vi "Main.vi"() -> ()   [LabVIEW 2017]
uses:
  <vilib>/Utility/miscctls.llb/LVRowAndColumnTypeDef.ctl
  flow_control/flow_queue_datatype.ctl
  <vilib>/Utility/miscctls.llb/LVPointTypeDef.ctl
  <vilib>/Utility/file.llb/Read Delimited Spreadsheet (string).vi
  <vilib>/Utility/file.llb/Write Delimited Spreadsheet (string).vi
panel:
  out "NG":string
  out "OK":string
  out "STATUS":string
  out "Edit Position":T1
  in  "Save Button":bool
  out "FILE":string[][](array[string])
  out "VISA resource name out":refnum<visa-resource-name>
  out "TESTING":bool
  in  "TEST Button":bool
  in  "Path":path
  out "DEFINE HEADER":string[][](array[string])
  out "Table":string[][](table)
  out "DEFINE IO":string[][](array[string])
  # "FT 4"
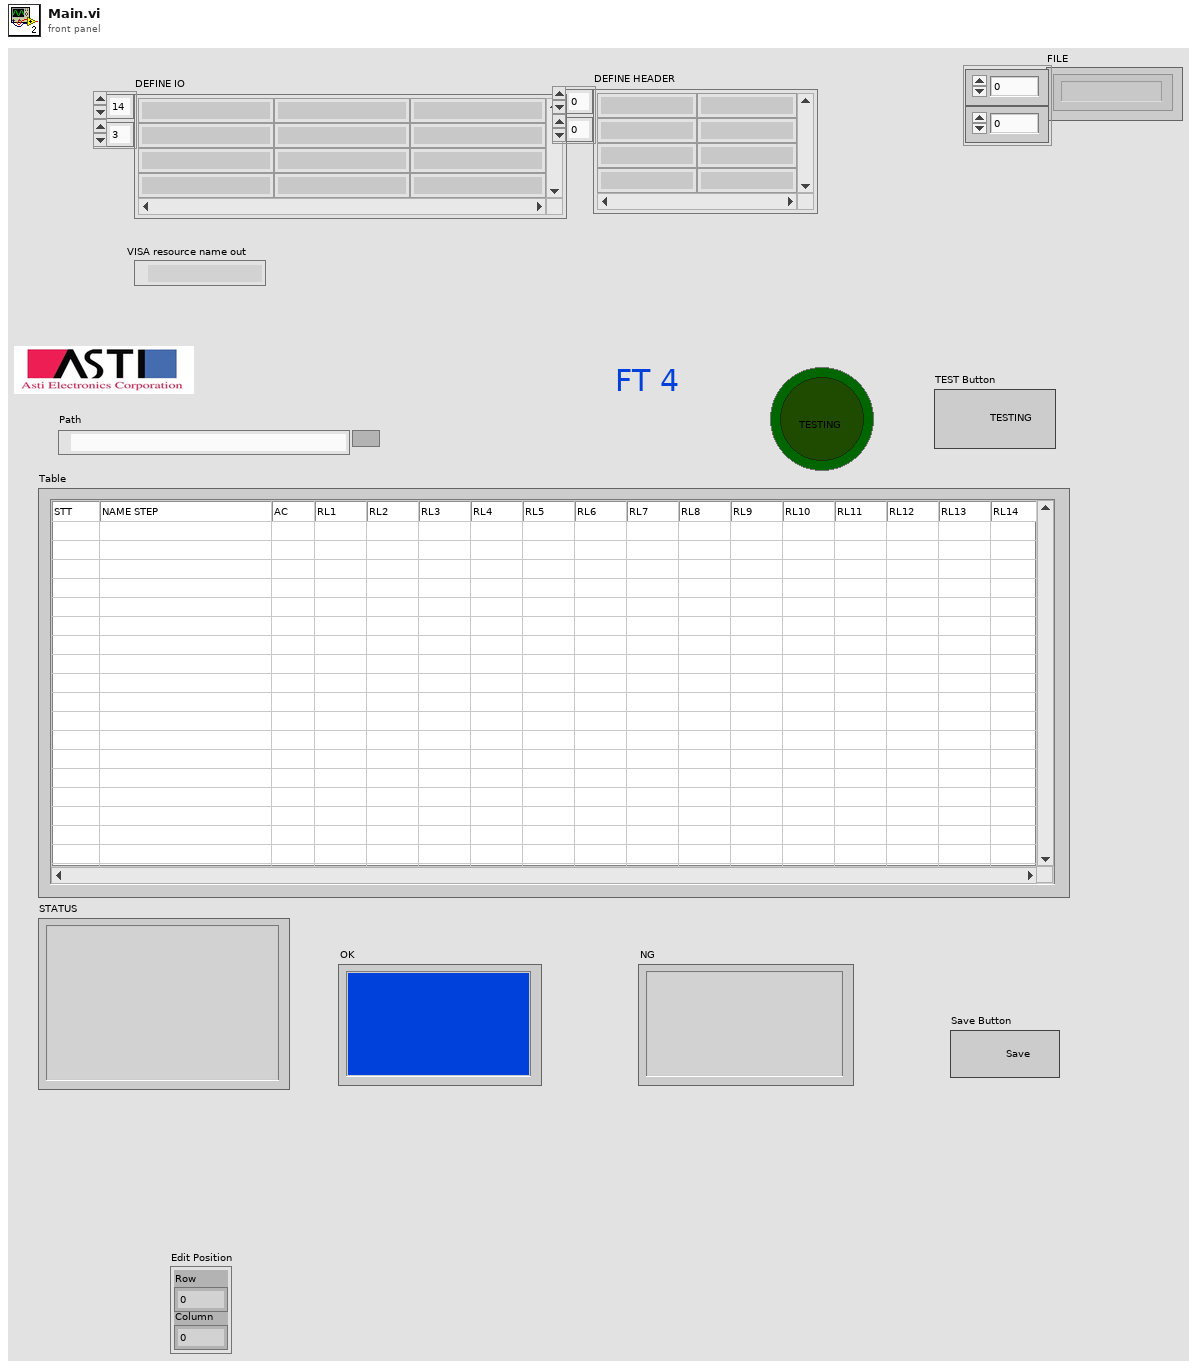
[diagram p1: front panel]
types:
  T1 = typedef "LVRowAndColumnTypeDef.ctl" = cluster{"Row":i32, "Column":i32}
  T2 = cluster{"queue name":string, "add \"initialize\" state":bool}[]
  T3 = typedef "flow_queue_datatype.ctl" = cluster{"command":string, "parameter":variant}
  T4 = typedef "LVPointTypeDef.ctl" = cluster{"Horizontal":i16, "Vertical":i16}
  T5 = cluster{"PORT":string, "BAUDRATE":string, "parity":string, "datab bits":string}
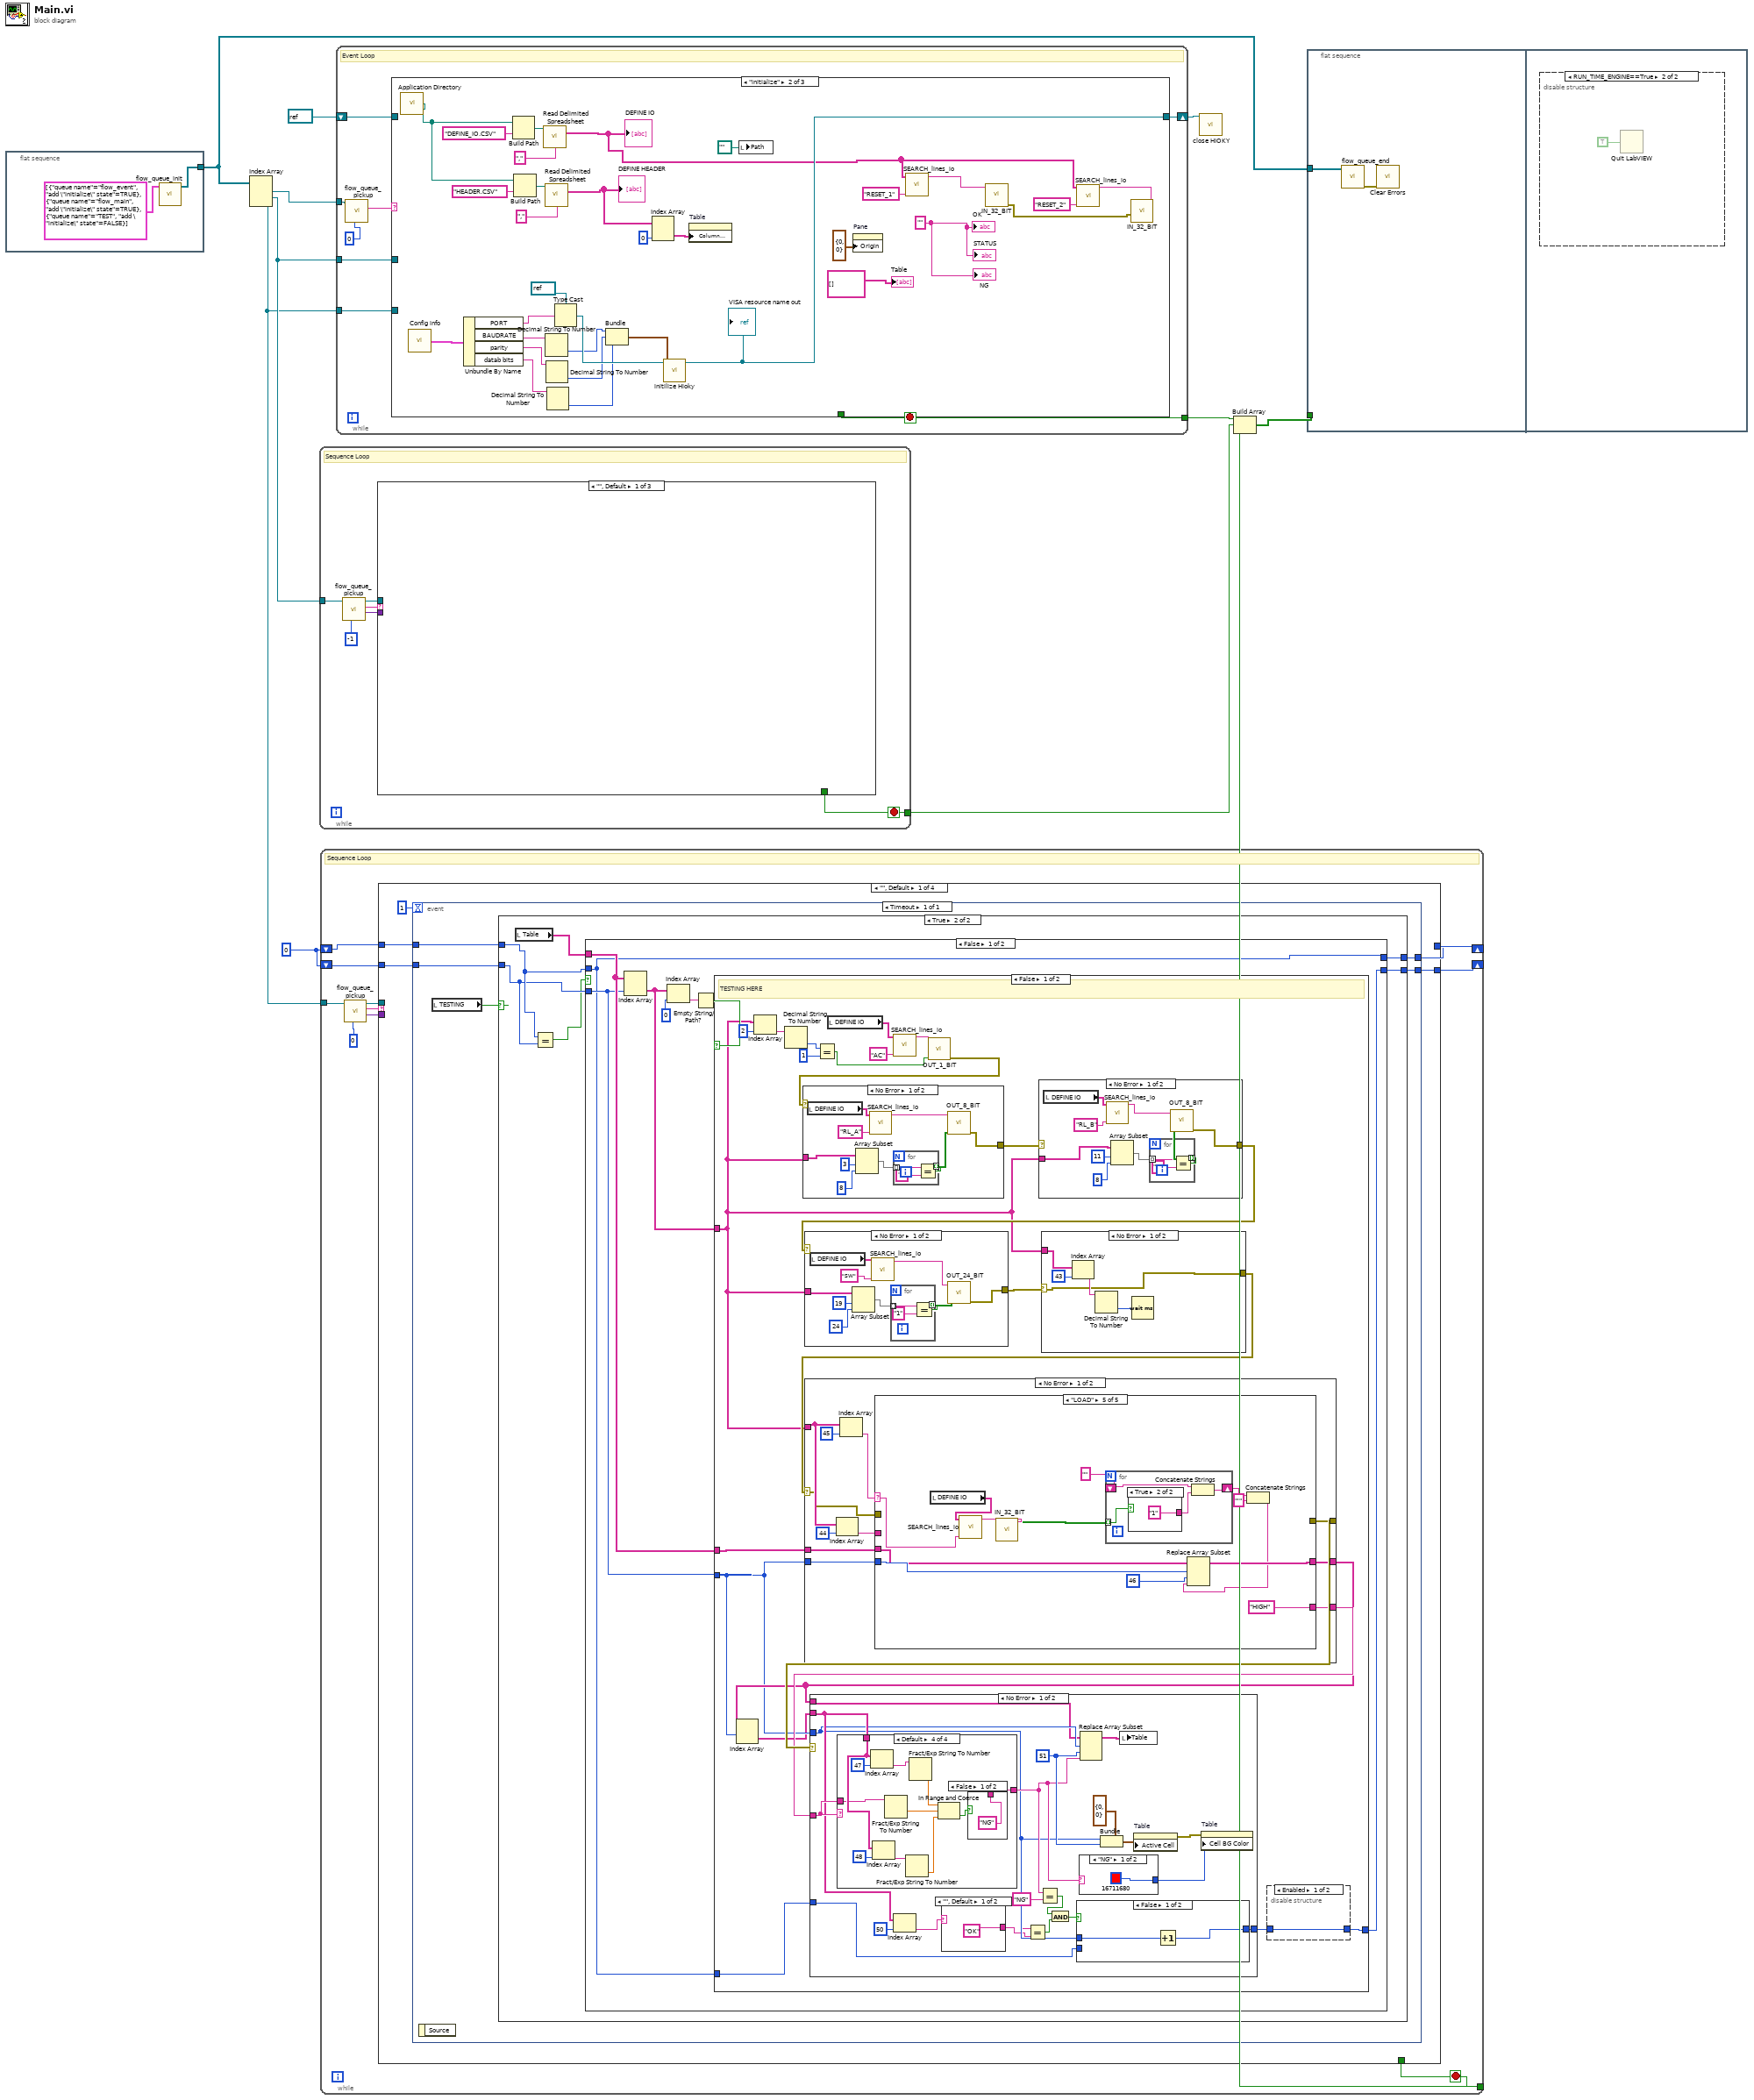
[diagram p0: block diagram]
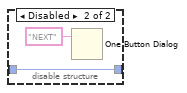
[diagram p3: hidden frame]
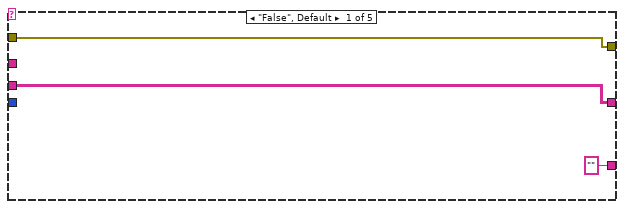
[diagram p4: hidden frame]
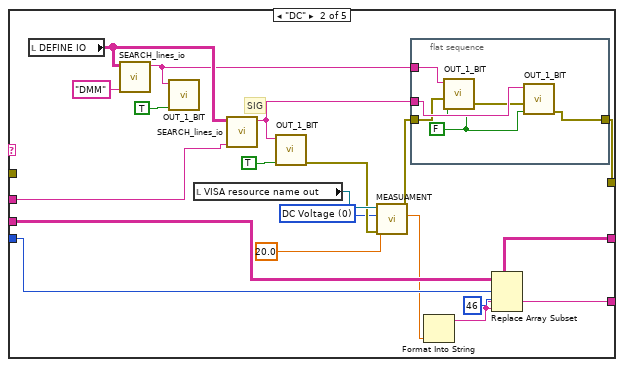
[diagram p5: hidden frame]
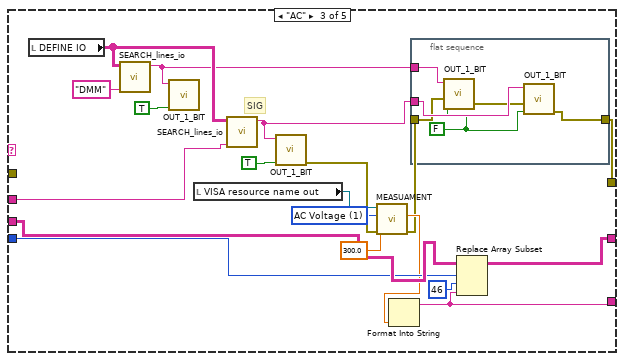
[diagram p6: hidden frame]
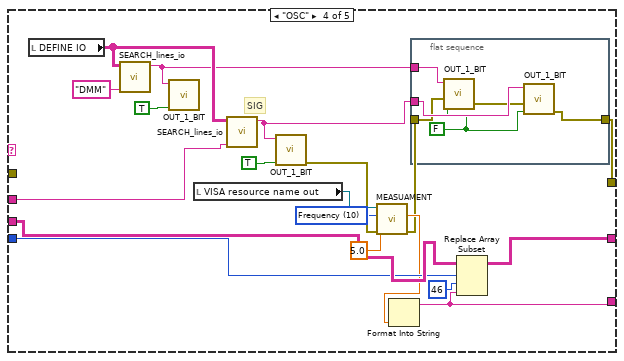
[diagram p7: hidden frame]
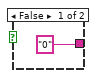
[diagram p8: hidden frame]
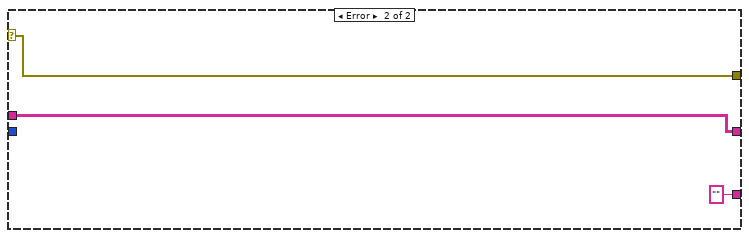
[diagram p9: hidden frame]
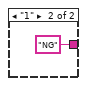
[diagram p11: hidden frame]
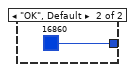
[diagram p12: hidden frame]
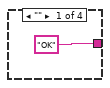
[diagram p13: hidden frame]
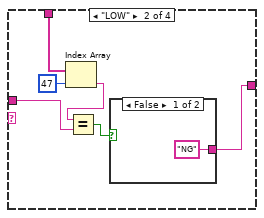
[diagram p14: hidden frame]
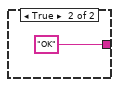
[diagram p15: hidden frame]
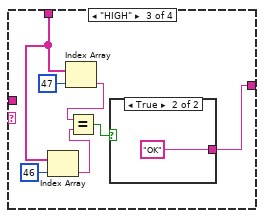
[diagram p16: hidden frame]
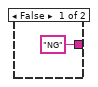
[diagram p17: hidden frame]
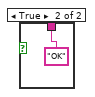
[diagram p18: hidden frame]
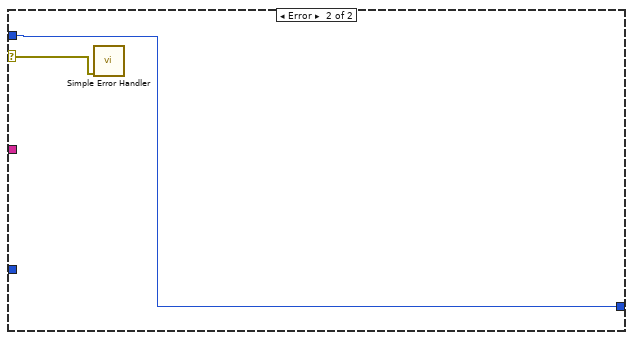
[diagram p19: hidden frame]
diagram:
  w2 = 0
  n1 = flat-sequence {
    tunnel: [w12] -> w9
    frame #0 {
      n2 = call "flow_queue_init.vi"("queue config"=T2 [{"queue name"="flow_event", "add \"initialize\" state"=TRUE}, {"queue name"="flow_main", "add \"initialize\" state"=TRUE}, {"queue name"="TEST", "add \"initialize\" state"=FALSE}]) -> ("flow_refnum"=w12:refnum<queue>[])  [unwired: 9 in, 1 out]
    }
  }
  n3 = Index Array(array=w9) -> (element #1=w11:refnum<queue>, element #2=w10:refnum<queue>, element #3=w3:refnum<queue>)  [unwired: 3 in]
  n4 = while {
    tunnel: w10 -> [w19]
    tunnel: [w15] -> w7
    stop <- w15 stop-if-true
    # "Sequence Loop"
    n5 = call "flow_queue_pickup.vi"("timeout"=-1, "queue in"=w19) -> ("parameter"=w14:variant, "command"=w18:string, "queue out"=w16:refnum<queue>)  [unwired: 5 in, 2 out]
    n6 = case shown="\"\", Default" w18 {
      tunnel: [_ TRUE _] -> w15
      tunnel: w16 -> [_ w20 _]
      tunnel: w14 -> [_ _ _]
      frame "", Default {
      }
      frame "end" {
        n7 = Flush Queue(queue=w20) -> ()  [unwired: 1 in, 3 out]
      }
      frame "initialize" {
      }
    }
  }
  n8 = while {
    tunnel: w3 -> [w31]
    tunnel: [w27] -> w1
    shift-right: [w25] -> _
    shift-left: w2 -> [w24]
    shift-right: [w23] -> _
    shift-left: w2 -> [w22]
    stop <- w27 stop-if-true
    # "Sequence Loop"
    n9 = call "flow_queue_pickup.vi"("timeout"=0, "queue in"=w31) -> ("parameter"=w26:variant, "command"=w30:string, "queue out"=w28:refnum<queue>)  [unwired: 5 in, 2 out]
    n10 = case shown="\"\", Default" w30 {
      tunnel: [_ _ TRUE _] -> w27
      tunnel: w28 -> [_ _ w340 _]
      tunnel: w26 -> [_ _ _ _]
      tunnel: [w33 w334 w339 w343] -> w25
      tunnel: w24 -> [w35 _ w339 w343]
      tunnel: [w32 0 ("index") w338 w342] -> w23
      tunnel: w22 -> [w34 _ w338 w342]
      frame "", Default {
        n11 = event shown="[0] Timeout" {
          selector: _ -> [_]
          dyn-events: _ -> [_]
          timeout: 1 -> [_]
          tunnel: w35 -> [w40]
          tunnel: w34 -> [w39]
          tunnel: [w38] -> w33
          tunnel: [w37] -> w32
          event Timeout {
            n12 = event-data() -> ()  [unwired: 1 in, 1 out]
            n13 = local read "TESTING"() -> (w41:bool)
            n14 = case shown="True" w41 {
              tunnel: w40 -> [w43 w47]
              tunnel: w39 -> [w42 w46]
              tunnel: [w43 w49] -> w38
              tunnel: [w42 w48] -> w37
              frame False {
              }
              frame True {
                n15 = local read "Table"() -> (w44:string[][])
                n16 = Equal?(x=w47, y=w46) -> (x = y?=w45:bool)
                n17 = case shown="False" w45 {
                  tunnel: w44 -> [w53 w305]
                  tunnel: w47 -> [w51 _]
                  tunnel: w46 -> [w52 _]
                  tunnel: [w51 w312] -> w49
                  tunnel: [w50 w312] -> w48
                  frame False {
                    n18 = Index Array "Index Array"(array=w53, index (row)=w52) -> (element=w54:string[])  [unwired: 1 in]
                    n19 = Index Array(array=w54, index=0) -> (element=w56:string)
                    n20 = Empty String/Path?(string/path=w56) -> (empty?=w55:bool)
                    n21 = case shown="False" w55 {
                      tunnel: w54 -> [w64 _]
                      tunnel: w53 -> [w70 _]
                      tunnel: w52 -> [w61 w300]
                      tunnel: w51 -> [w63 _]
                      tunnel: [w58 w300] -> w50
                      frame False {
                        # "TESTING HERE"
                        n22 = Index Array(array=w64, index=2) -> (element=w79:string)
                        n23 = Decimal String To Number(string=w79) -> (number=w78:i32)  [unwired: 2 in, 1 out]
                        n24 = Equal?(x=w78, y=1) -> (x = y?=w66:bool)
                        n25 = local read "DEFINE IO"() -> (w69:string[][])
                        n26 = call "SEARCH_lines_io.vi"("IN str"="AC", "Array define"=w69) -> ("OUT lines"=w67:string)  [unwired: 9 in]
                        n27 = call "OUT_1_BIT.vi"("data"=w66, "String"=w67) -> ("error out"=w76:errorcluster)  [unwired: 9 in]
                        n28 = case shown="No Error" w76 {
                          selector: w76 -> [_ w299]
                          tunnel: [w295 w299] -> w75
                          tunnel: w64 -> [w294 _]
                          frame No Error {
                            n29 = local read "DEFINE IO"() -> (w287:string[][])
                            n30 = Array Subset(array=w294, index=3, length=8 ("index")) -> (w291:string[])
                            n31 = call "SEARCH_lines_io.vi"("IN str"="RL_A", "Array define"=w287) -> ("OUT lines"=w288:string)  [unwired: 9 in]
                            n32 = for {
                              tunnel: w291 -> [w298] mode=indexing
                              tunnel: [w296] -> w290 mode=indexing
                              n33 = Equal?(x=w298, y="1") -> (x = y?=w296:bool)
                            }
                            n34 = call "OUT_8_BIT.vi"("data"=w290, "String"=w288) -> ("error out"=w295:errorcluster)  [unwired: 9 in]
                          }
                          frame Error {
                          }
                        }
                        n35 = case shown="No Error" w75 {
                          selector: w75 -> [_ w286]
                          tunnel: [w282 w286] -> w74
                          tunnel: w64 -> [w281 _]
                          frame No Error {
                            n36 = local read "DEFINE IO"() -> (w274:string[][])
                            n37 = call "SEARCH_lines_io.vi"("IN str"="RL_B" ("element"), "Array define"=w274) -> ("OUT lines"=w275:string)  [unwired: 9 in]
                            n38 = Array Subset(array=w281, index=11, length=8 ("index")) -> (w278:string[])
                            n39 = for {
                              tunnel: w278 -> [w285] mode=indexing
                              tunnel: [w283] -> w277 mode=indexing
                              n40 = Equal?(x=w285, y="1") -> (x = y?=w283:bool)
                            }
                            n41 = call "OUT_8_BIT.vi"("data"=w277, "String"=w275) -> ("error out"=w282:errorcluster)  [unwired: 9 in]
                          }
                          frame Error {
                          }
                        }
                        n42 = case shown="No Error" w74 {
                          selector: w74 -> [_ w273]
                          tunnel: [w269 w273] -> w73
                          tunnel: w64 -> [w268 _]
                          frame No Error {
                            n43 = local read "DEFINE IO"() -> (w262:string[][])
                            n44 = Array Subset(array=w268, index=19, length=24 ("index")) -> (w265:string[])
                            n45 = call "SEARCH_lines_io.vi"("IN str"="SW" ("element"), "Array define"=w262) -> ("OUT lines"=w261:string)  [unwired: 9 in]
                            n46 = for {
                              tunnel: w265 -> [w272] mode=indexing
                              tunnel: [w270] -> w264 mode=indexing
                              n47 = Equal?(x=w272, y="1") -> (x = y?=w270:bool)
                            }
                            n48 = call "OUT_24_BIT.vi"("Array"=w264, "String"=w261) -> ("error out"=w269:errorcluster)  [unwired: 9 in]
                          }
                          frame Error {
                          }
                        }
                        n49 = case shown="No Error" w73 {
                          selector: w73 -> [w255 w260]
                          tunnel: w64 -> [w259 _]
                          tunnel: [w255 w260] -> w72
                          frame No Error {
                            n50 = Index Array(array=w259, index=43) -> (element=w257:string)
                            n51 = Decimal String To Number(string=w257) -> (number=w256:i32)  [unwired: 2 in, 1 out]
                            n52 = Wait (ms)(milliseconds to wait=w256) -> ()  [unwired: 1 out]
                          }
                          frame Error {
                          }
                        }
                        n53 = case shown="No Error" w72 {
                          selector: w72 -> [w86 w194]
                          tunnel: w64 -> [w91 _]
                          tunnel: w70 -> [w89 w192]
                          tunnel: w61 -> [w88 _]
                          tunnel: [w87 w194] -> w71
                          tunnel: [w85 ""] -> w65
                          tunnel: [w84 w192] -> w62
                          frame No Error {
                            n54 = Index Array(array=w91, index=44) -> (element=w90:string)
                            n55 = Index Array(array=w91, index=45) -> (element=w93:string)
                            n56 = case shown="\"LOAD\"" w93 {
                              selector: w93 -> [_ _ _ _ w180]
                              tunnel: w90 -> [_ w112 w137 w162 _]
                              tunnel: w89 -> [w95 w109 w134 w159 w181]
                              tunnel: w88 -> [_ w108 w133 w158 w182]
                              tunnel: [w97 w105 w130 w155 _] -> w87
                              tunnel: w86 -> [w97 _ _ _ _]
                              tunnel: ["" w101 w126 w151 "HIGH"] -> w85
                              tunnel: [w95 w100 w125 w150 w176] -> w84
                              frame "False", Default {
                              }
                              frame "DC" {
                                w99 = u16 0 items=["DC Voltage", "AC Voltage", "2 - Wire Resistance", "2 -Wire Resistance low power", "4 - Wire Resistance", "4- Wire Resistance low power", "DC Current", "AC Current", "CLAMP DC", "CLAMP AC", "Frequency", "Continuity", "Diode Checking"] ("Function (0: DC Voltage)")
                                # "SIG"
                                n57 = local read "DEFINE IO"() -> (w113:string[][])
                                n58 = call "SEARCH_lines_io.vi"("IN str"="DMM", "Array define"=w113) -> ("OUT lines"=w103:string)  [unwired: 9 in]
                                n59 = call "OUT_1_BIT.vi"("data"=TRUE, "String"=w103) -> ()  [unwired: 9 in, 1 out]
                                n60 = local read "VISA resource name out"() -> (w111:refnum<visa-resource-name>)
                                n61 = call "SEARCH_lines_io.vi"("IN str"=w112, "Array define"=w113) -> ("OUT lines"=w102:string)  [unwired: 9 in]
                                n62 = call "OUT_1_BIT.vi"("data"=TRUE, "String"=w102) -> ("error out"=w106:errorcluster)  [unwired: 9 in]
                                n63 = call "MEASUAMENT.vi"("error in (no error)"=w106, "Manual Range (1.00)"=20.0, "Function (0: DC Voltage)"=w99, "VISA resource name"=w111) -> ("error out"=w104:errorcluster, "Measurement"=w107:dbl)  [unwired: 5 in, 1 out]
                                n64 = flat-sequence {
                                tunnel: [w117] -> w105
                                tunnel: w104 -> [w118]
                                tunnel: w103 -> [w122]
                                tunnel: w102 -> [w121]
                                frame #0 {
                                w119 = FALSE ("data")
                                n65 = call "OUT_1_BIT.vi"("data"=w119, "error in"=w118, "String"=w122) -> ("error out"=w120:errorcluster)  [unwired: 8 in]
                                n66 = call "OUT_1_BIT.vi"("data"=w119, "error in"=w120, "String"=w121) -> ("error out"=w117:errorcluster)  [unwired: 8 in]
                                }
                                }
                                n67 = Format Into String(w107) -> (resulting string=w101:string)  [unwired: 3 in, 1 out]
                                n68 = Replace Array Subset "Replace Array Subset"(array=w109, new element=w101, index (row)=w108, index (col)=46 ("index")) -> (w100:string[][])
                              }
                              frame "AC" {
                                w124 = u16 1 items=["DC Voltage", "AC Voltage", "2 - Wire Resistance", "2 -Wire Resistance low power", "4 - Wire Resistance", "4- Wire Resistance low power", "DC Current", "AC Current", "CLAMP DC", "CLAMP AC", "Frequency", "Continuity", "Diode Checking"] ("Function (0: DC Voltage)")
                                # "SIG"
                                n69 = local read "DEFINE IO"() -> (w138:string[][])
                                n70 = call "SEARCH_lines_io.vi"("IN str"="DMM", "Array define"=w138) -> ("OUT lines"=w128:string)  [unwired: 9 in]
                                n71 = call "OUT_1_BIT.vi"("data"=TRUE, "String"=w128) -> ()  [unwired: 9 in, 1 out]
                                n72 = local read "VISA resource name out"() -> (w136:refnum<visa-resource-name>)
                                n73 = call "SEARCH_lines_io.vi"("IN str"=w137, "Array define"=w138) -> ("OUT lines"=w127:string)  [unwired: 9 in]
                                n74 = call "OUT_1_BIT.vi"("data"=TRUE, "String"=w127) -> ("error out"=w131:errorcluster)  [unwired: 9 in]
                                n75 = call "MEASUAMENT.vi"("error in (no error)"=w131, "Manual Range (1.00)"=300.0, "Function (0: DC Voltage)"=w124, "VISA resource name"=w136) -> ("error out"=w129:errorcluster, "Measurement"=w132:dbl)  [unwired: 5 in, 1 out]
                                n76 = Format Into String(w132) -> (resulting string=w126:string)  [unwired: 3 in, 1 out]
                                n77 = flat-sequence {
                                tunnel: [w142] -> w130
                                tunnel: w129 -> [w143]
                                tunnel: w128 -> [w147]
                                tunnel: w127 -> [w146]
                                frame #0 {
                                w144 = FALSE ("data")
                                n78 = call "OUT_1_BIT.vi"("data"=w144, "error in"=w143, "String"=w147) -> ("error out"=w145:errorcluster)  [unwired: 8 in]
                                n79 = call "OUT_1_BIT.vi"("data"=w144, "error in"=w145, "String"=w146) -> ("error out"=w142:errorcluster)  [unwired: 8 in]
                                }
                                }
                                n80 = Replace Array Subset "Replace Array Subset"(array=w134, new element=w126, index (row)=w133, index (col)=46 ("index")) -> (w125:string[][])
                              }
                              frame "OSC" {
                                w149 = u16 10 items=["DC Voltage", "AC Voltage", "2 - Wire Resistance", "2 -Wire Resistance low power", "4 - Wire Resistance", "4- Wire Resistance low power", "DC Current", "AC Current", "CLAMP DC", "CLAMP AC", "Frequency", "Continuity", "Diode Checking"] ("Function (0: DC Voltage)")
                                # "SIG"
                                n81 = local read "DEFINE IO"() -> (w163:string[][])
                                n82 = call "SEARCH_lines_io.vi"("IN str"="DMM", "Array define"=w163) -> ("OUT lines"=w153:string)  [unwired: 9 in]
                                n83 = call "OUT_1_BIT.vi"("data"=TRUE, "String"=w153) -> ()  [unwired: 9 in, 1 out]
                                n84 = local read "VISA resource name out"() -> (w161:refnum<visa-resource-name>)
                                n85 = call "SEARCH_lines_io.vi"("IN str"=w162, "Array define"=w163) -> ("OUT lines"=w152:string)  [unwired: 9 in]
                                n86 = call "OUT_1_BIT.vi"("data"=TRUE, "String"=w152) -> ("error out"=w156:errorcluster)  [unwired: 9 in]
                                n87 = call "MEASUAMENT.vi"("error in (no error)"=w156, "Manual Range (1.00)"=5.0, "Function (0: DC Voltage)"=w149, "VISA resource name"=w161) -> ("error out"=w154:errorcluster, "Measurement"=w157:dbl)  [unwired: 5 in, 1 out]
                                n88 = Format Into String(w157) -> (resulting string=w151:string)  [unwired: 3 in, 1 out]
                                n89 = flat-sequence {
                                tunnel: [w167] -> w155
                                tunnel: w154 -> [w168]
                                tunnel: w153 -> [w172]
                                tunnel: w152 -> [w171]
                                frame #0 {
                                w169 = FALSE ("data")
                                n90 = call "OUT_1_BIT.vi"("data"=w169, "error in"=w168, "String"=w172) -> ("error out"=w170:errorcluster)  [unwired: 8 in]
                                n91 = call "OUT_1_BIT.vi"("data"=w169, "error in"=w170, "String"=w171) -> ("error out"=w167:errorcluster)  [unwired: 8 in]
                                }
                                }
                                n92 = Replace Array Subset "Replace Array Subset"(array=w159, new element=w151, index (row)=w158, index (col)=46 ("index")) -> (w150:string[][])
                              }
                              frame "LOAD" {
                                n93 = local read "DEFINE IO"() -> (w185:string[][])
                                n94 = call "SEARCH_lines_io.vi"("IN str"=w180, "Array define"=w185) -> ("OUT lines"=w184:string)  [unwired: 9 in]
                                n95 = call "IN_32_BIT.vi"("String"=w184) -> ("data"=w179:bool[])  [unwired: 9 in, 1 out]
                                n96 = for {
                                tunnel: w179 -> [w189] mode=indexing
                                shift-right: [w187] -> w175
                                shift-left: "" -> [w186]
                                n97 = case shown="True" w189 {
                                tunnel: ["0" "1"] -> w188
                                frame False {
                                }
                                frame True {
                                }
                                }
                                n98 = Concatenate Strings(w186, w188) -> (w187:string)
                                }
                                n99 = Concatenate Strings(w175, "'" ("string")) -> (w174:string)
                                n100 = Replace Array Subset "Replace Array Subset"(array=w181, new element=w174, index (row)=w182, index (col)=46 ("index")) -> (w176:string[][])
                              }
                            }
                          }
                          frame Error {
                          }
                        }
                        n101 = Index Array(array=w62, index (row)=w61) -> (element=w60:string[])  [unwired: 1 in]
                        n102 = case shown="No Error" w71 {
                          selector: w71 -> [_ w254]
                          tunnel: w61 -> [w203 w253]
                          tunnel: w65 -> [w208 _]
                          tunnel: w60 -> [w206 _]
                          tunnel: w63 -> [w201 _]
                          tunnel: [w202 w253] -> w59
                          tunnel: w62 -> [w195 _]
                          frame No Error {
                            w200 = "NG" ("y")
                            w211 = 51 ("index")
                            n103 = case shown="Default" w208 {
                              tunnel: w206 -> [_ w227 w232 w248]
                              tunnel: w208 -> [_ w225 _ w245]
                              tunnel: ["OK" ("new element/subarray") w224 w235 w240] -> w204
                              frame "" {
                              }
                              frame "LOW" {
                                n104 = Index Array(array=w227, index=47) -> (element=w226:string)
                                n105 = Equal?(x=w226, y=w225) -> (x = y?=w223:bool)
                                n106 = case shown="False" w223 {
                                tunnel: ["NG" "OK"] -> w224
                                frame False {
                                }
                                frame True {
                                }
                                }
                              }
                              frame "HIGH" {
                                n107 = Index Array(array=w232, index=46) -> (element=w231:string)
                                n108 = Index Array(array=w232, index=47) -> (element=w236:string)
                                n109 = Equal?(x=w236, y=w231) -> (x = y?=w234:bool)
                                n110 = case shown="True" w234 {
                                tunnel: ["NG" "OK"] -> w235
                                frame False {
                                }
                                frame True {
                                }
                                }
                              }
                              frame Default {
                                n111 = Index Array(array=w248, index=47) -> (element=w247:string)
                                n112 = Index Array(array=w248, index=48) -> (element=w246:string)
                                n113 = Fract/Exp String To Number(string=w245) -> (number=w242:dbl)  [unwired: 3 in, 1 out]
                                n114 = Fract/Exp String To Number(string=w246) -> (number=w243:dbl)  [unwired: 3 in, 1 out]
                                n115 = Fract/Exp String To Number(string=w247) -> (number=w244:dbl)  [unwired: 3 in, 1 out]
                                n116 = In Range and Coerce(upper limit=w244, x=w242, lower limit=w243) -> (In Range?=w241:bool)  [unwired: 1 out]
                                n117 = case shown="False" w241 {
                                tunnel: ["NG" "OK"] -> w240
                                frame False {
                                }
                                frame True {
                                }
                                }
                              }
                            }
                            n118 = Index Array(array=w206, index=50) -> (element=w205:string)
                            n119 = case shown="\"\", Default" w205 {
                              tunnel: ["OK" "NG"] -> w199
                              frame "", Default {
                              }
                              frame "1" {
                              }
                            }
                            n120 = Equal?(x=w200, y=w199) -> (x = y?=w197:bool)
                            n121 = Equal?(x=w204, y=w200) -> (x = y?=w198:bool)
                            n122 = And(x=w198, y=w197) -> (x .and. y?=w196:bool)
                            n123 = case shown="False" w196 {
                              tunnel: w203 -> [w216 _]
                              tunnel: [w215 w217] -> w202
                              tunnel: w201 -> [_ w217]
                              frame False {
                                n124 = Increment(x=w216) -> (x+1=w215:i32)
                              }
                              frame True {
                              }
                            }
                            n125 = case shown="\"NG\"" w204 {
                              tunnel: [u32 16711680 u32 16860] -> w209
                              frame "NG" {
                              }
                              frame "OK", Default {
                              }
                            }
                            n126 = Replace Array Subset "Replace Array Subset"(array=w195, new element=w204, index (row)=w203, index (col)=w211) -> (w214:string[][])
                            n127 = Bundle(cluster=T1 {"Row"=0, "Column"=0} ("Active Cell:Active Cell"), "Row"=w203, "Column"=w211) -> (w212:T1)
                            n128 = local write "Table"(w214) -> ()
                            n129 = property on="Table" class="Tbl (strict)"("Active Cell"=w212) -> (error out=w210:errorcluster)  [unwired: 2 in, 1 out]
                            n130 = property on="Table" class="Tbl (strict)"(error in=w210, "Cell BG Color"=w209) -> ()  [unwired: 1 in, 2 out]
                          }
                          frame Error {
                            n131 = call <vilib>:"Simple Error Handler.vi"("error in (no error)"=w254) -> ()  [unwired: 4 in, 5 out]
                          }
                        }
                        n132 = disable-structure shown="Enabled" {
                          disable-tunnel: w59 -> [w81 w83]
                          disable-tunnel: [w81 w83] -> w58
                          frame Enabled {
                          }
                          frame Disabled {
                            n133 = One Button Dialog(message="NEXT") -> ()  [unwired: 1 in, 1 out]
                          }
                        }
                      }
                      frame True {
                      }
                    }
                  }
                  frame True {
                    w312 = 0
                    n134 = Index Array(array=w305, index (col)=51 ("disabled index (col)")) -> (element=w303:string[])  [unwired: 1 in]
                    n135 = local write "TESTING"(FALSE ("TESTING")) -> ()
                    n136 = local read "DEFINE IO"() -> (w308:string[][])
                    n137 = for {
                      tunnel: w303 -> [w329] mode=indexing
                      tunnel: [w326] -> w302 mode=indexing
                      n138 = Equal?(x=w329, y="OK") -> (x = y?=w327:bool)
                      n139 = case shown="True" w327 {
                        tunnel: [FALSE TRUE] -> w326
                        frame False {
                        }
                        frame True {
                        }
                      }
                    }
                    n140 = call "SEARCH_lines_io.vi"("IN str"="RESET_1", "Array define"=w308) -> ("OUT lines"=w310:string)  [unwired: 9 in]
                    n141 = call "IN_32_BIT.vi"("String"=w310) -> ("error out"=w306:errorcluster)  [unwired: 9 in, 1 out]
                    n142 = call "SEARCH_lines_io.vi"("IN str"="RESET_2", "Array define"=w308) -> ("OUT lines"=w307:string)  [unwired: 9 in]
                    n143 = And Array Elements(Boolean array=w302) -> (logical AND=w301:bool)
                    n144 = call "IN_32_BIT.vi"("error in"=w306, "String"=w307) -> ()  [unwired: 8 in, 2 out]
                    n145 = case shown="False" w301 {
                      frame False {
                        w314 = u32 16711680
                        n146 = local read "NG"() -> (w319:string)
                        n147 = Decimal String To Number(string=w319) -> (number=w318:i32)  [unwired: 2 in, 1 out]
                        n148 = local write "STATUS"("NG" ("STATUS")) -> ()
                        n149 = property on="STATUS" class="Str"("Text.TextColor"=w314) -> ()  [unwired: 2 in, 2 out]
                        n150 = Increment(x=w318) -> (x+1=w317:i32)
                        n151 = property on="NG" class="Str"("Text.TextColor"=w314) -> ()  [unwired: 2 in, 2 out]
                        n152 = Number To Decimal String(number=w317) -> (decimal integer string=w316:string)  [unwired: 1 in]
                        n153 = local write "NG"(w316) -> ()
                      }
                      frame True {
                        w320 = u32 16860
                        n154 = local read "OK"() -> (w324:string)
                        n155 = Decimal String To Number(string=w324) -> (number=w323:i32)  [unwired: 2 in, 1 out]
                        n156 = local write "STATUS"("OK" ("STATUS")) -> ()
                        n157 = property on="STATUS" class="Str"("Text.TextColor"=w320) -> ()  [unwired: 2 in, 2 out]
                        n158 = Increment(x=w323) -> (x+1=w322:i32)
                        n159 = property on="OK" class="Str"("Text.BGColor"=w320) -> ()  [unwired: 2 in, 2 out]
                        n160 = Number To Decimal String(number=w322) -> (decimal integer string=w321:string)  [unwired: 1 in]
                        n161 = local write "OK"(w321) -> ()
                      }
                    }
                  }
                }
              }
            }
          }
        }
      }
      frame "TEST" {
        n162 = local read "Table"() -> (w332:string[][])
        n163 = local write "TESTING"(TRUE ("TESTING")) -> ()
        n164 = Array Size(array=w332) -> (size(s)=w336:i32[])
        n165 = Index Array(array=w336, index=0) -> (element=w334:i32)
      }
      frame "end" {
        n166 = Flush Queue(queue=w340) -> ()  [unwired: 1 in, 3 out]
      }
      frame "initialize" {
      }
    }
  }
  n167 = while {
    tunnel: w11 -> [w351]
    tunnel: w10 -> [w348]
    tunnel: [w347] -> w8
    shift-right: [w346] -> w4
    shift-left: refnum<visa-resource-name> refnum ("VISA resource name out") -> [w345]
    tunnel: w3 -> [w344]
    stop <- w347 stop-if-true
    # "Event Loop"
    n168 = call "flow_queue_pickup.vi"("timeout"=0, "queue in"=w351) -> ("command"=w350:string)  [unwired: 5 in, 4 out]
    n169 = case shown="\"initialize\"" w350 {
      tunnel: w348 -> [w355 _ w441]
      tunnel: [w354 _ TRUE] -> w347
      tunnel: [w353 w423 w438] -> w346
      tunnel: w345 -> [w353 _ w438]
      tunnel: w344 -> [w352 _ _]
      frame "", Default {
        n170 = event shown="[1] \"Path\": Value Change" {
          selector: _ -> [_ _ _ _ _ _]
          dyn-events: _ -> [_ _ _ _ _ _]
          timeout: _ -> [_ _ _ _ _ _]
          tunnel: w355 -> [_ _ _ w392 _ _]
          tunnel: [_ _ _ w391 _ _] -> w354
          tunnel: w352 -> [_ _ w373 w388 _ _]
          event Timeout {
            n171 = event-data() -> ()  [unwired: 1 in, 3 out]
          }
          event "Path": Value Change {
            w360 = ""
            n172 = event-data() -> ()  [unwired: 1 in, 6 out]
            n173 = call-poly <vilib>:"Read Delimited Spreadsheet.vi"("file path (dialog if empty)"="Path", "delimiter (\\t)"="," ("delimiter (\\t)")) -> ("all rows"=w362:string[][])  [unwired: 8 in, 5 out]
            n174 = local write "NG"(w360) -> ()
            n175 = local write "OK"(w360) -> ()
            n176 = local write "STATUS"(w360) -> ()
            n177 = Array Subset(array=w362, index (row)=1 ("index")) -> (w356:string[][])  [unwired: 3 in]
            "FILE" <- w356
            n178 = Array Size(array=w356) -> (size(s)=w359:i32[])
            n179 = Index Array(array=w359, index=0) -> (element=w358:i32)
            n180 = local write "Table"(w356) -> ()
            n181 = for {
              N: w358 -> [_]
              i -> [w369]
              n182 = Bundle By Name(cluster=T1 {"Row"=0, "Column"=0} ("Active Cell:Active Cell"), "Row"=w369, "Column"=51 ("disabled index (col)")) -> (w366:T1)
              n183 = property on="Table" class="Tbl (strict)"("Active Cell"=w366) -> (error out=w368:errorcluster)  [unwired: 2 in, 1 out]
              n184 = property on="Table" class="Tbl (strict)"(error in=w368, "Cell BG Color"=u32 16448250) -> ()  [unwired: 1 in, 2 out]
            }
          }
          event "TEST Button": Value Change {
            n185 = event-data() -> ()  [unwired: 1 in, 6 out]
            n186 = flat-sequence {
              tunnel: [w375] -> w372
              tunnel: [w374] -> w371
              frame #0 {
                n187 = invoke on="Table" class="Tbl (strict)" method="Reinit To Default"() -> ()  [unwired: 3 in, 3 out]
                n188 = local read "FILE"() -> (w374:string[][])
                n189 = Empty Array?(array=w374) -> (empty?=w375:bool)
              }
            }
            n190 = case shown="False" w372 {
              tunnel: w373 -> [_ w380]
              tunnel: w371 -> [_ w379]
              frame True {
              }
              frame False {
                n191 = Array Size(array=w379) -> (size(s)=w378:i32[])
                n192 = Index Array(array=w378, index=0) -> (element=w376:i32)
                n193 = for {
                  N: w376 -> [_]
                  i -> [w386]
                  n194 = Bundle By Name(cluster=T1 {"Row"=0, "Column"=0} ("Active Cell:Active Cell"), "Row"=w386, "Column"=51 ("disabled index (col)")) -> (w383:T1)
                  n195 = property on="Table" class="Tbl (strict)"("Active Cell"=w383) -> (error out=w385:errorcluster)  [unwired: 2 in, 1 out]
                  n196 = property on="Table" class="Tbl (strict)"(error in=w385, "Cell BG Color"=u32 16448250) -> ()  [unwired: 1 in, 2 out]
                }
                n197 = call "flow_queue_add.vi"("data"=T3 {"command"="TEST", "parameter"=variant}, "queue in"=w380) -> ()  [unwired: 8 in, 2 out]
                n198 = local write "Table"(w379) -> ()
              }
            }
          }
          event Panel Close? {
            n199 = event-data() -> ()  [unwired: 1 in, 4 out]
            n200 = Two Button Dialog(message="Do you want to exit ?") -> (T button?=w390:bool)  [unwired: 2 in]
            n201 = case shown="True" w390 {
              tunnel: w392 -> [_ w398]
              tunnel: [_ TRUE] -> w391
              tunnel: w388 -> [_ w395]
              frame False {
              }
              frame True {
                n202 = call "flow_queue_add.vi"("data"=T3 {"command"="end", "parameter"=variant}, "queue in"=w398) -> ()  [unwired: 8 in, 2 out]
                n203 = call "flow_queue_add.vi"("data"=T3 {"command"="end", "parameter"=variant}, "queue in"=w395) -> ()  [unwired: 8 in, 2 out]
              }
            }
            n204 = event-data("Discard?"=TRUE) -> ()  [unwired: 1 in, 1 out]
          }
          event "Save Button": Value Change {
            n205 = event-data() -> ()  [unwired: 1 in, 6 out]
            n206 = local read "Table"() -> (w400:string[][])
            n207 = Empty Array?(array=w400) -> (empty?=w399:bool)
            n208 = case shown="False" w399 {
              tunnel: w400 -> [w402 _]
              frame False {
                n209 = call-poly <vilib>:"Write Delimited Spreadsheet.vi"("2D data"=w402, "delimiter (\\t)"="," ("delimiter (\\t)")) -> ()  [unwired: 12 in, 2 out]
              }
              frame True {
              }
            }
          }
          event "Table": Mouse Down {
            n210 = event-data() -> ()  [unwired: 1 in, 8 out]
            n211 = local read "Path"() -> (w404:path)
            n212 = Empty String/Path?(string/path=w404) -> (empty?=w403:bool)
            n213 = case shown="False" w403 {
              frame False {
                n214 = property on="Table" class="Tbl (strict)"() -> ("EditPos"=→"Edit Position":T1)  [unwired: 2 in, 2 out]
              }
              frame True {
              }
            }
          }
        }
      }
      frame "initialize" {
        w407 = ""
        n215 = call <vilib>:"Application Directory.vi"() -> ("Application Directory"=w419:path)
        n216 = call "Config info.vi"() -> ("info com main"=w434:T5)  [unwired: 13 in, 2 out]
        n217 = Unbundle By Name(w434) -> ("PORT"=w433:string, "BAUDRATE"=w430:string, "parity"=w429:string, "datab bits"=w428:string)
        n218 = Build Path(base path=w419, name or relative path="DEFINE_IO.CSV") -> (appended path=w436:path)
        n219 = Build Path(base path=w419, name or relative path="HEADER.CSV") -> (appended path=w421:path)
        n220 = call-poly <vilib>:"Read Delimited Spreadsheet.vi"("file path (dialog if empty)"=w436, "delimiter (\\t)"="," ("delimiter (\\t)")) -> ("all rows"=w409:string[][])  [unwired: 8 in, 5 out]
        "DEFINE IO" <- w409
        n221 = call-poly <vilib>:"Read Delimited Spreadsheet.vi"("file path (dialog if empty)"=w421, "delimiter (\\t)"="," ("delimiter (\\t)")) -> ("all rows"=w418:string[][])  [unwired: 8 in, 5 out]
        "DEFINE HEADER" <- w418
        n222 = Decimal String To Number(string=w430) -> (number=w427:i32)  [unwired: 2 in, 1 out]
        n223 = Decimal String To Number(string=w429) -> (number=w426:i32)  [unwired: 2 in, 1 out]
        n224 = Decimal String To Number(string=w428) -> (number=w425:i32)  [unwired: 2 in, 1 out]
        n225 = Type Cast(type=refnum<visa-resource-name> refnum ("VISA resource name"), x=w433) -> (*(type *) &x=w431:refnum<visa-resource-name>)
        n226 = Bundle(w427, w426, w425) -> (w424:cluster{i32, i32, i32})  [unwired: 1 in]
        n227 = Index Array(array=w418, index (col)=0 ("disabled index (col)")) -> (element=w416:string[])  [unwired: 1 in]
        n228 = call "initilize Hioky.vi"("Serial Configuration"=w424, "VISA resource name"=w431) -> ("VISA resource name out"=w423:refnum<visa-resource-name>)  [unwired: 8 in, 1 out]
        "VISA resource name out" <- w423
        n229 = property on="Table" class="Tbl (strict)"("Column Headers[]"=w416) -> ()  [unwired: 2 in, 2 out]
        n230 = local write "Path"(path "" ("Path")) -> ()
        n231 = property on="Pane" class="Pane"("Origin"=T4 {"Horizontal"=0, "Vertical"=0}) -> ()  [unwired: 2 in, 2 out]
        n232 = call "SEARCH_lines_io.vi"("IN str"="RESET_1", "Array define"=w409) -> ("OUT lines"=w414:string)  [unwired: 9 in]
        n233 = call "IN_32_BIT.vi"("String"=w414) -> ("error out"=w412:errorcluster)  [unwired: 9 in, 1 out]
        n234 = call "SEARCH_lines_io.vi"("IN str"="RESET_2", "Array define"=w409) -> ("OUT lines"=w413:string)  [unwired: 9 in]
        n235 = call "IN_32_BIT.vi"("error in"=w412, "String"=w413) -> ()  [unwired: 8 in, 2 out]
        "Table" <- string[][] []
        "STATUS" <- w407
        "OK" <- w407
        "NG" <- w407
      }
      frame "end" {
        n236 = call "flow_queue_add.vi"("data"=T3 {"command"="end", "parameter"=variant}, "queue in"=w441) -> ()  [unwired: 8 in, 2 out]
      }
    }
  }
  n237 = call "close HIOKY.vi"("VISA resource name"=w4) -> ()  [unwired: 10 in, 1 out]
  n238 = Build Array(w8, w7, w1) -> (w6:bool[])
  n239 = flat-sequence {
    tunnel: w9 -> [w443]
    tunnel: w6 -> [_]
    frame #0 {
      n240 = call "flow_queue_end.vi"("flow_refnum"=w443) -> ("error out"=w442:errorcluster)  [unwired: 10 in]
      n241 = call <vilib>:"Clear Errors.vi"("error in (no error)"=w442) -> ()  [unwired: 5 in, 2 out]
    }
    frame #1 {
      n242 = disable-structure shown="RUN_TIME_ENGINE==True" {
        frame condition #0 (active) {
        }
        frame condition #1 {
          n243 = Quit LabVIEW(quit? (T)=TRUE ("終了?（T）")) -> ()
        }
      }
    }
  }
